vi "PmacCoordMotorDef.vi"(3 "Motor Number i32 (1-8) (1)":i32=1 min=1 max=8, 4 "Coord Number i32 (1-8) (1)":i32=1 min=1 max=8, 5 "Device Number i32 (0)":i32) -> (0 "Coord Defined Bool (F)":bool, 1 "Coord Scale Dbl (1.0)":dbl format="%.2f", 2 "Coord Definition String":string)   [LabVIEW 2020]
doc: "Query PMAC for the definition of Motor Number in Coord Number. If the motor is not defined in the specified CS Coord Definition is \"Encoder\", Coord Scale = 1.0, and Coord Defined is FALSE. If the motor is defined in the specified CS Coord Defined is TRUE, Coord Scale is the encoder to CS unit scale factor, and Coord Definition is the definition (e.g. \"#1->16000X\")."
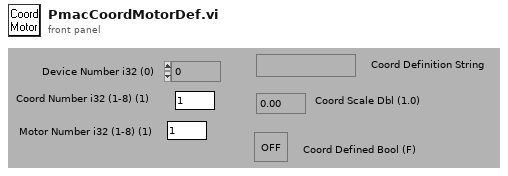
[diagram p1: front panel]
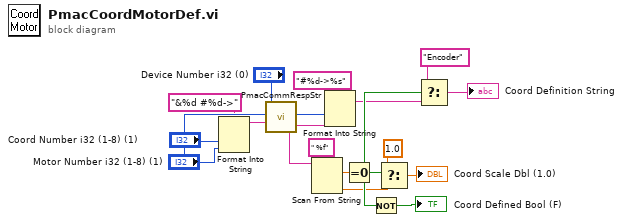
[diagram p0: block diagram]
diagram:
  n1 = Format Into String(format string="&%d #%d->", "Coord Number i32 (1-8) (1)", "Motor Number i32 (1-8) (1)") -> (resulting string=w8:string)  [unwired: 2 in, 1 out]
  n2 = call "PmacCommRespStr.vi"("Command String"=w8, "Device Number i32 (0)"="Device Number i32 (0)") -> ("Response String (\"\")"=w6:string)  [unwired: 1 out]
  n3 = Scan From String(format string=" %f", input string=w6) -> (output 1=w10:dbl)  [unwired: 2 in, 4 out]
  n4 = Format Into String(format string="#%d->%s", "Motor Number i32 (1-8) (1)", w6) -> (resulting string=w3:string)  [unwired: 2 in, 1 out]
  n5 = Equal To 0?(x=w10) -> (x = 0?=w12:bool)
  n6 = Not(x=w12) -> (.not. x?=→"Coord Defined Bool (F)":bool)
  n7 = Select(t=1.0, s=w12, f=w10) -> (s? t:f=→"Coord Scale Dbl (1.0)":dbl)
  n8 = Select(t="Encoder", s=w12, f=w3) -> (s? t:f=→"Coord Definition String":string)
